vi "GUI Interlock Tester-teardown.vi"(8 "Self Test Button":refnum<vi>, 9 "Power Off Button":refnum<vi>, 10 "Power On Button":refnum<vi>, 11 "test case ID":string) -> (3 "result":bool)   [LabVIEW 2018]
doc: "The teardown VI should be executed after the VI under test in the harness VI. In this VI you can evaluate the outputs of the VI under test.\n\nSee the Help Document for more information. (<b>Help</b> > <b>IncQuery Labs</b> > <b>InstaCoverage</b> > <b>InstaCoverage Help...</b>)"
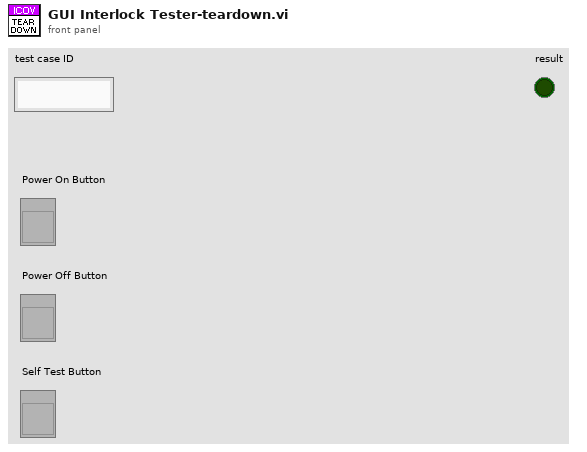
[diagram p1: front panel]
types:
  T1 = enum8{"Enabled", "Disabled", "Disabled and Grayed Out"}
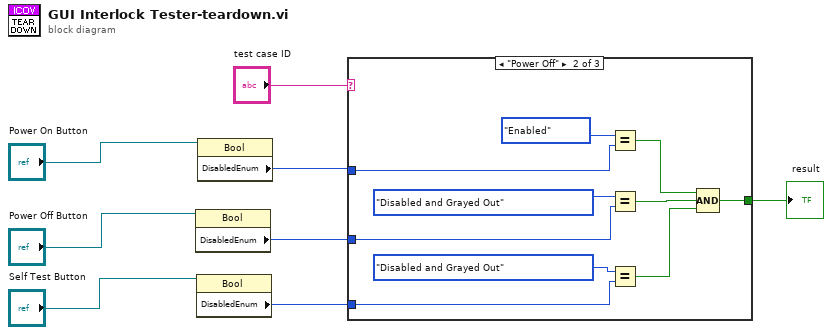
[diagram p0: block diagram]
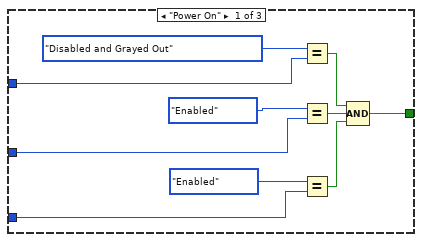
[diagram p2: hidden frame]
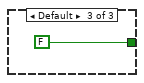
[diagram p3: hidden frame]
diagram:
  n1 = property class="Bool"(reference="Power Off Button") -> ("DisabledEnum"=w5:T1)  [unwired: 1 in, 2 out]
  n2 = property class="Bool"(reference="Self Test Button") -> ("DisabledEnum"=w4:T1)  [unwired: 1 in, 2 out]
  n3 = property class="Bool"(reference="Power On Button") -> ("DisabledEnum"=w6:T1)  [unwired: 1 in, 2 out]
  n4 = case shown="\"Power Off\"" "test case ID" {
    tunnel: [w12 w19 FALSE] -> w7
    tunnel: w6 -> [w17 w27 _]
    tunnel: w5 -> [w15 w25 _]
    tunnel: w4 -> [w13 w23 _]
    frame "Power On" {
      n5 = Equal?(x=T1."Disabled and Grayed Out" ("Disabled"), y=w17) -> (x = y?=w11:bool)
      n6 = Equal?(x=T1."Enabled" ("Disabled"), y=w15) -> (x = y?=w10:bool)
      n7 = Equal?(x=T1."Enabled" ("Disabled"), y=w13) -> (x = y?=w9:bool)
      n8 = Compound Arithmetic op=AND(w11, w10, w9) -> (w12:bool)
    }
    frame "Power Off" {
      n9 = Equal?(x=T1."Enabled" ("Disabled"), y=w27) -> (x = y?=w22:bool)
      n10 = Equal?(x=T1."Disabled and Grayed Out" ("Disabled"), y=w25) -> (x = y?=w21:bool)
      n11 = Equal?(x=T1."Disabled and Grayed Out" ("Disabled"), y=w23) -> (x = y?=w20:bool)
      n12 = Compound Arithmetic op=AND(w22, w21, w20) -> (w19:bool)
    }
    frame Default {
    }
  }
  "result" <- w7
